vi "SubVI_Prescan Trace.vi"(0 "VISA in":refnum<visa-resource-name>, 1 "Cable 1":T5, 2 "Cable 2":T4, 3 "Cable 3":T3, 5 "Antenna":T6, 7 "Attenuator":T2, 9 "Amplifier":T1=enum."10K-2GHz ME813", 11 "error in (no error)":errorcluster, 12 "Trace 2D array input":dbl[][](array[numeric])) -> (4 "VISA out":refnum<visa-resource-name>, 6 "Start Frequency":dbl, 8 "Stop Frequency":dbl, 10 "Corrected amplitude 1D array":dbl[](array[numeric]), 13 "Completed Result Table":dbl[][](array[numeric]), 14 "Corrected System Trace":cluster{dbl[], "x+y":dbl[]}, 15 "error out":errorcluster)   [LabVIEW 2016]
doc: "This VI generate corrected plot of measurement system adding up antenna factor, cable loss, attenuation and amplification along the way."
uses:
  Antenna.ctl
  Cable 1.ctl
  Cable 2.ctl
  Cable 3.ctl
  Attenuator.ctl
  Amplifier.ctl
panel:
  out "AmplifierX_1D array":dbl[](array[numeric])
  out "AmplifierY_1D array":dbl[](array[numeric]) format="%_6g"
  out "AttenuatorX_1D array":dbl[](array[numeric])
  out "AttenuatorY_1D array":dbl[](array[numeric]) format="%_6g"
  out "Cable3X_1D array":dbl[](array[numeric])
  out "Cable3Y_1D array":dbl[](array[numeric]) format="%_6g"
  out "Cable2X_1D array":dbl[](array[numeric])
  out "Cable2Y_1D array":dbl[](array[numeric]) format="%_6g"
  out "Cable1Y_1D array":dbl[](array[numeric]) format="%_6g"
  out "Cable1X_1D array":dbl[](array[numeric])
  out "Antenna X 1D array":dbl[](array[numeric])
  out "Antenna Y 1D array":dbl[](array[numeric]) format="%_6g"
  out "Nuber of Points":i32
  out "XY Graph":cluster{dbl[], "x+y":dbl[]}(graph)
  out "Corrected 2D array":dbl[][](array[numeric])
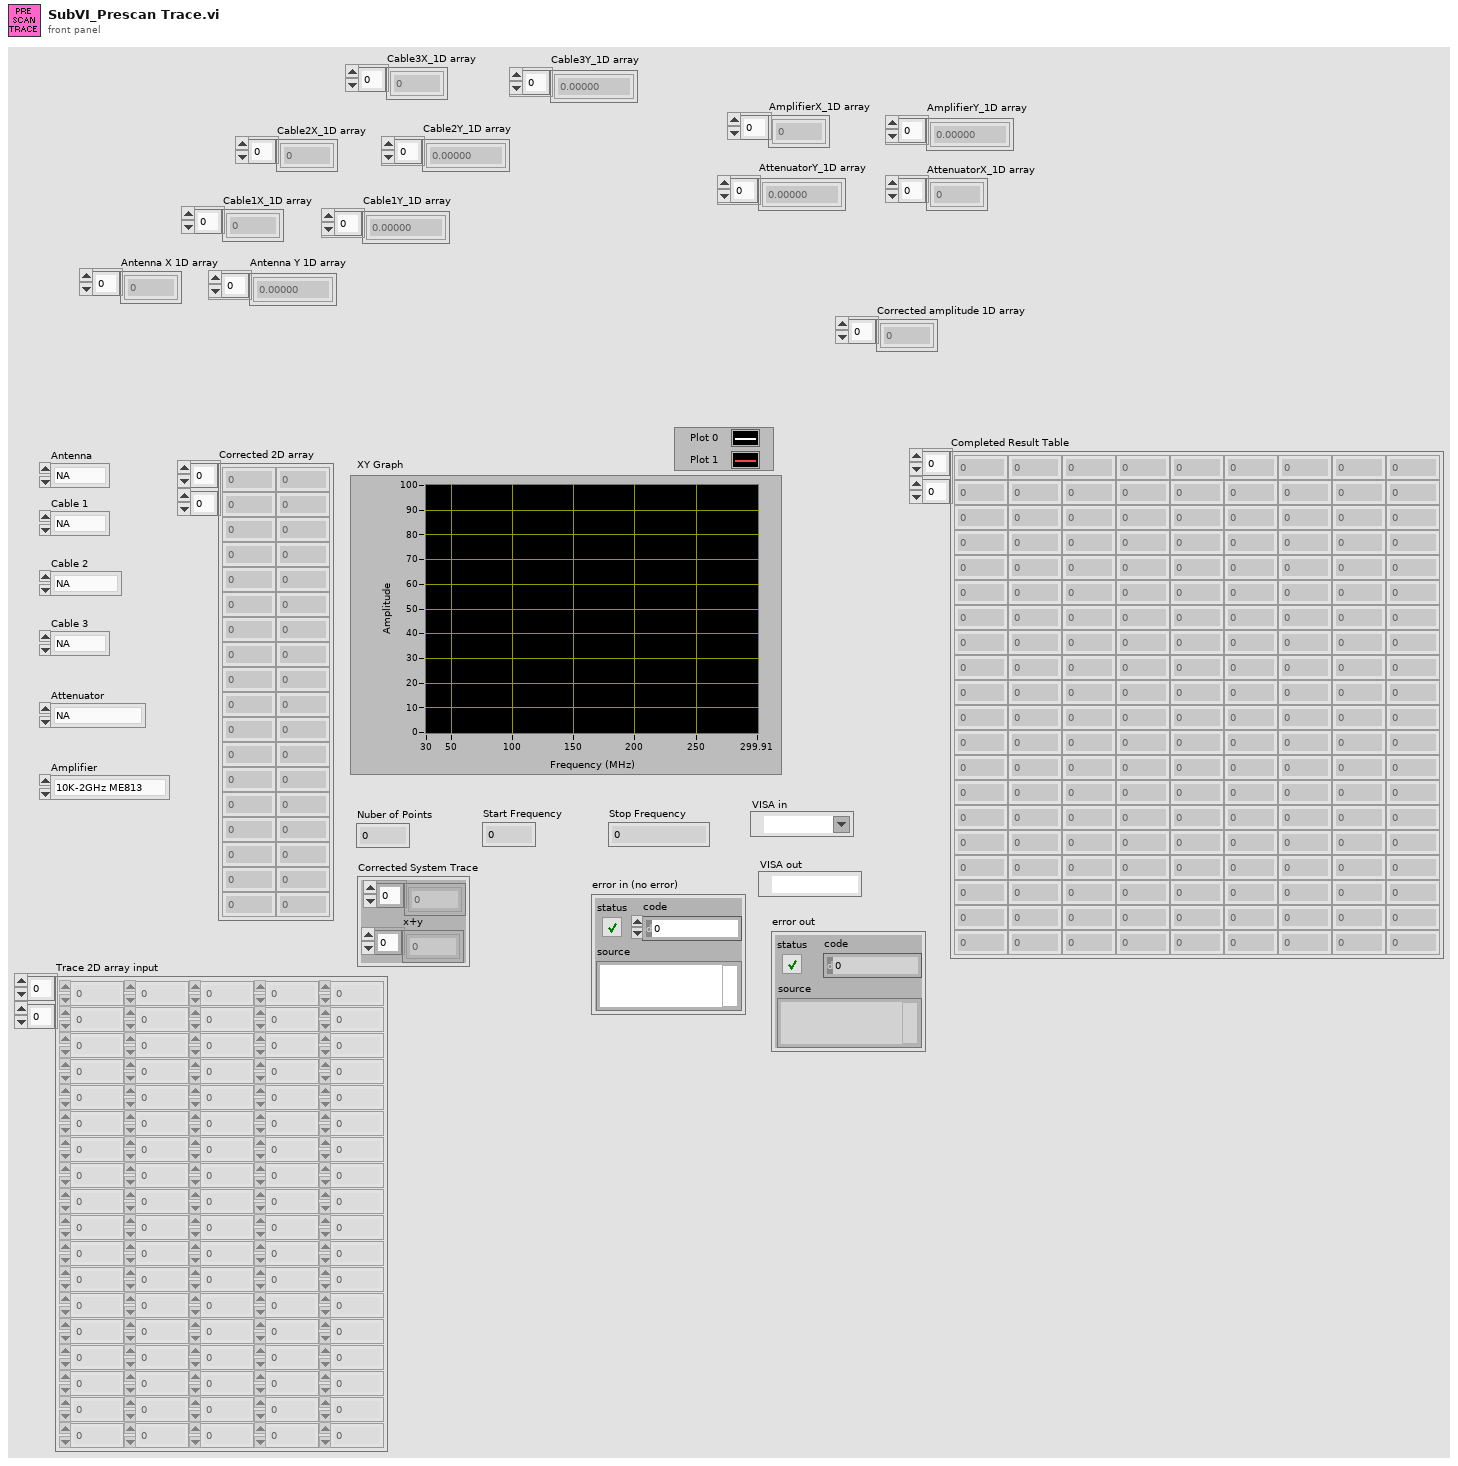
[diagram p1: front panel]
types:
  T1 = typedef "Amplifier.ctl" = enum16{"NA", "10K-2GHz ME813", "500M-18GHz ME1241"}
  T2 = typedef "Attenuator.ctl" = enum16{"NA", "6dB-ME811"}
  T3 = typedef "Cable 3.ctl" = enum16{"NA", "ME1244", "ME1245", "ME1249"}
  T4 = typedef "Cable 2.ctl" = enum16{"NA", "ME1244", "ME1245", "ME1249"}
  T5 = typedef "Cable 1.ctl" = enum16{"NA", "ME1244", "ME1245", "ME1249"}
  T6 = typedef "Antenna.ctl" = enum16{"NA", "ME828 Biconical", "ME1284 Periodical"}
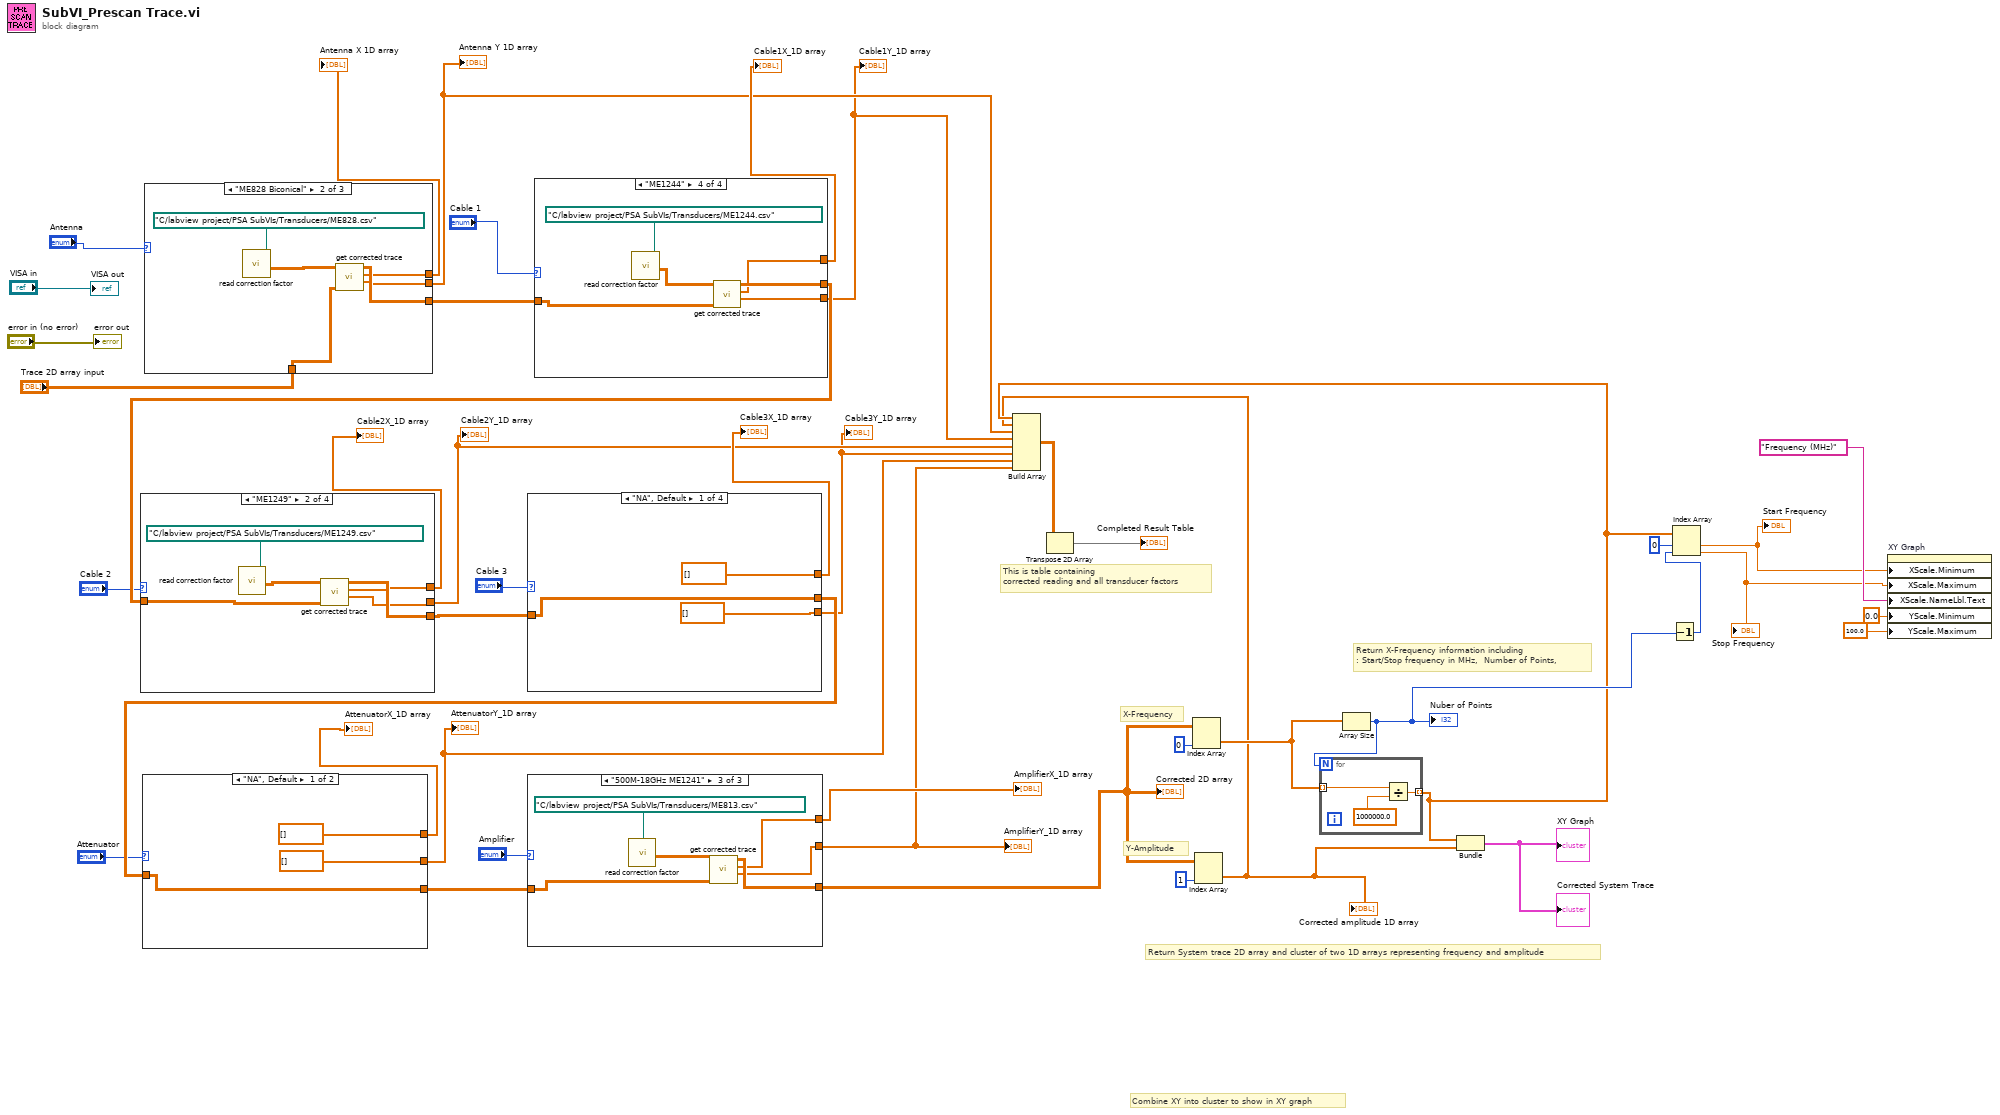
[diagram p0: block diagram]
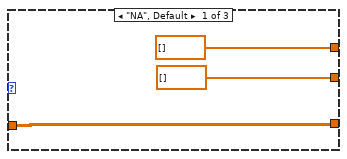
[diagram p2: hidden frame]
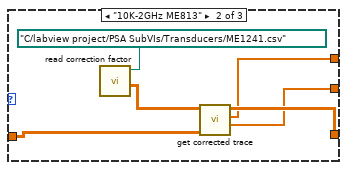
[diagram p3: hidden frame]
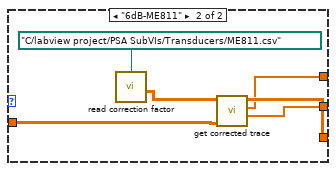
[diagram p4: hidden frame]
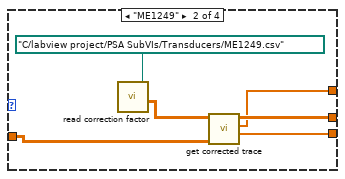
[diagram p5: hidden frame]
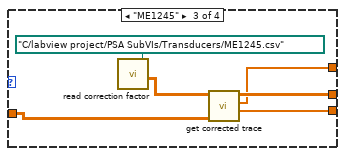
[diagram p6: hidden frame]
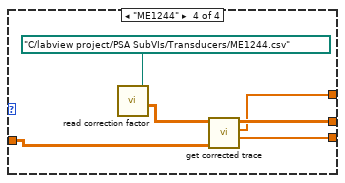
[diagram p7: hidden frame]
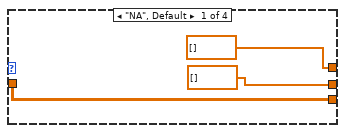
[diagram p8: hidden frame]
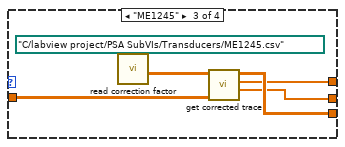
[diagram p9: hidden frame]
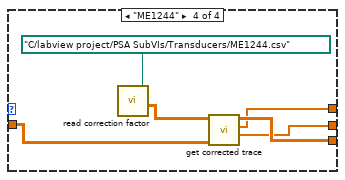
[diagram p10: hidden frame]
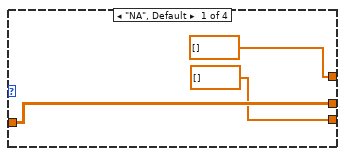
[diagram p11: hidden frame]
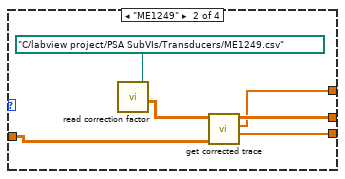
[diagram p12: hidden frame]
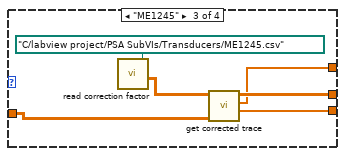
[diagram p13: hidden frame]
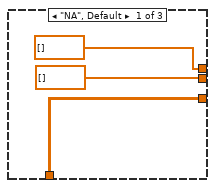
[diagram p14: hidden frame]
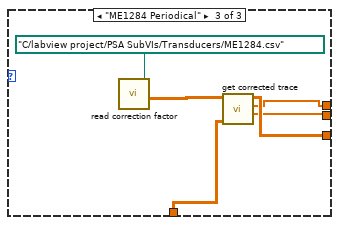
[diagram p15: hidden frame]
diagram:
  # "This is table containing \ncorrected reading and all transducer factors"
  # "Return System trace 2D array and cluster of two 1D arrays representing frequency and amplitude"
  # "Combine XY into cluster to show in XY graph"
  # "Return X-Frequency information including\n: Start/Stop frequency in MHz,  Number of Points,"
  # "Y-Amplitude"
  # "X-Frequency"
  n1 = case shown="\"ME828 Biconical\"" "Antenna" {
    tunnel: "Trace 2D array input" -> [w46 w49 w55]
    tunnel: [w46 w50 w56] -> w43
    tunnel: [dbl[] [] ("xi used") w48 w54] -> w17
    tunnel: [dbl[] [] ("xi used") w47 w53] -> w7
    frame "NA", Default {
    }
    frame "ME828 Biconical" {
      n2 = call "read correction factor.vi"("Path"=path "C:/labview project/PSA SubVIs/Transducers/ME828.csv") -> ("Output Array"=w52:dbl[][])  [unwired: 7 in, 3 out]
      n3 = call "get corrected trace.vi"("Trace 2D array"=w49, "Transducer 2D array"=w52) -> ("yi"=w47:dbl[], "xi used"=w48:dbl[], "x+y"=w50:dbl[][])  [unwired: 7 in]
    }
    frame "ME1284 Periodical" {
      n4 = call "read correction factor.vi"("Path"=path "C:/labview project/PSA SubVIs/Transducers/ME1284.csv") -> ("Output Array"=w58:dbl[][])  [unwired: 7 in, 3 out]
      n5 = call "get corrected trace.vi"("Trace 2D array"=w55, "Transducer 2D array"=w58) -> ("yi"=w53:dbl[], "xi used"=w54:dbl[], "x+y"=w56:dbl[][])  [unwired: 7 in]
    }
  }
  "Antenna Y 1D array" <- w7
  "Antenna X 1D array" <- w17
  n6 = case shown="\"ME1244\"" "Cable 1" {
    tunnel: w43 -> [w61 w65 w71 w77]
    tunnel: [w61 w64 w70 w76] -> w42
    tunnel: [dbl[] [] ("xi used") w63 w69 w75] -> w16
    tunnel: [dbl[] [] ("xi used") w62 w68 w74] -> w6
    frame "NA", Default {
    }
    frame "ME1249" {
      n7 = call "read correction factor.vi"("Path"=path "C:/labview project/PSA SubVIs/Transducers/ME1249.csv") -> ("Output Array"=w66:dbl[][])  [unwired: 7 in, 3 out]
      n8 = call "get corrected trace.vi"("Trace 2D array"=w65, "Transducer 2D array"=w66) -> ("yi"=w62:dbl[], "xi used"=w63:dbl[], "x+y"=w64:dbl[][])  [unwired: 7 in]
    }
    frame "ME1245" {
      n9 = call "read correction factor.vi"("Path"=path "C:/labview project/PSA SubVIs/Transducers/ME1245.csv") -> ("Output Array"=w72:dbl[][])  [unwired: 7 in, 3 out]
      n10 = call "get corrected trace.vi"("Trace 2D array"=w71, "Transducer 2D array"=w72) -> ("yi"=w68:dbl[], "xi used"=w69:dbl[], "x+y"=w70:dbl[][])  [unwired: 7 in]
    }
    frame "ME1244" {
      n11 = call "read correction factor.vi"("Path"=path "C:/labview project/PSA SubVIs/Transducers/ME1244.csv") -> ("Output Array"=w78:dbl[][])  [unwired: 7 in, 3 out]
      n12 = call "get corrected trace.vi"("Trace 2D array"=w77, "Transducer 2D array"=w78) -> ("yi"=w74:dbl[], "xi used"=w75:dbl[], "x+y"=w76:dbl[][])  [unwired: 7 in]
    }
  }
  "Cable1X_1D array" <- w16
  "Cable1Y_1D array" <- w6
  n13 = case shown="\"ME1249\"" "Cable 2" {
    tunnel: w42 -> [w82 w86 w92 w98]
    tunnel: [w82 w85 w91 w97] -> w41
    tunnel: [dbl[] [] ("xi used") w84 w90 w96] -> w15
    tunnel: [dbl[] [] ("xi used") w83 w89 w95] -> w5
    frame "NA", Default {
    }
    frame "ME1249" {
      n14 = call "read correction factor.vi"("Path"=path "C:/labview project/PSA SubVIs/Transducers/ME1249.csv") -> ("Output Array"=w87:dbl[][])  [unwired: 7 in, 3 out]
      n15 = call "get corrected trace.vi"("Trace 2D array"=w86, "Transducer 2D array"=w87) -> ("yi"=w83:dbl[], "xi used"=w84:dbl[], "x+y"=w85:dbl[][])  [unwired: 7 in]
    }
    frame "ME1245" {
      n16 = call "read correction factor.vi"("Path"=path "C:/labview project/PSA SubVIs/Transducers/ME1245.csv") -> ("Output Array"=w93:dbl[][])  [unwired: 7 in, 3 out]
      n17 = call "get corrected trace.vi"("Trace 2D array"=w92, "Transducer 2D array"=w93) -> ("yi"=w89:dbl[], "xi used"=w90:dbl[], "x+y"=w91:dbl[][])  [unwired: 7 in]
    }
    frame "ME1244" {
      n18 = call "read correction factor.vi"("Path"=path "C:/labview project/PSA SubVIs/Transducers/ME1244.csv") -> ("Output Array"=w99:dbl[][])  [unwired: 7 in, 3 out]
      n19 = call "get corrected trace.vi"("Trace 2D array"=w98, "Transducer 2D array"=w99) -> ("yi"=w95:dbl[], "xi used"=w96:dbl[], "x+y"=w97:dbl[][])  [unwired: 7 in]
    }
  }
  "Cable2X_1D array" <- w15
  "Cable2Y_1D array" <- w5
  n20 = case shown="\"NA\", Default" "Cable 3" {
    tunnel: w41 -> [w103 w107 w113 w119]
    tunnel: [w103 w106 w112 w118] -> w40
    tunnel: [dbl[] [] ("xi used") w105 w111 w117] -> w14
    tunnel: [dbl[] [] ("xi used") w104 w110 w116] -> w4
    frame "NA", Default {
    }
    frame "ME1249" {
      n21 = call "read correction factor.vi"("Path"=path "C:/labview project/PSA SubVIs/Transducers/ME1249.csv") -> ("Output Array"=w108:dbl[][])  [unwired: 7 in, 3 out]
      n22 = call "get corrected trace.vi"("Trace 2D array"=w107, "Transducer 2D array"=w108) -> ("yi"=w104:dbl[], "xi used"=w105:dbl[], "x+y"=w106:dbl[][])  [unwired: 7 in]
    }
    frame "ME1245" {
      n23 = call "read correction factor.vi"("Path"=path "C:/labview project/PSA SubVIs/Transducers/ME1245.csv") -> ("Output Array"=w114:dbl[][])  [unwired: 7 in, 3 out]
      n24 = call "get corrected trace.vi"("Trace 2D array"=w113, "Transducer 2D array"=w114) -> ("yi"=w110:dbl[], "xi used"=w111:dbl[], "x+y"=w112:dbl[][])  [unwired: 7 in]
    }
    frame "ME1244" {
      n25 = call "read correction factor.vi"("Path"=path "C:/labview project/PSA SubVIs/Transducers/ME1244.csv") -> ("Output Array"=w120:dbl[][])  [unwired: 7 in, 3 out]
      n26 = call "get corrected trace.vi"("Trace 2D array"=w119, "Transducer 2D array"=w120) -> ("yi"=w116:dbl[], "xi used"=w117:dbl[], "x+y"=w118:dbl[][])  [unwired: 7 in]
    }
  }
  "Cable3X_1D array" <- w14
  "Cable3Y_1D array" <- w4
  n27 = case shown="\"NA\", Default" "Attenuator" {
    tunnel: w40 -> [w124 w128]
    tunnel: [w124 w127] -> w39
    tunnel: [dbl[] [] ("xi used") w126] -> w13
    tunnel: [dbl[] [] ("xi used") w125] -> w3
    frame "NA", Default {
    }
    frame "6dB-ME811" {
      n28 = call "read correction factor.vi"("Path"=path "C:/labview project/PSA SubVIs/Transducers/ME811.csv") -> ("Output Array"=w129:dbl[][])  [unwired: 7 in, 3 out]
      n29 = call "get corrected trace.vi"("Trace 2D array"=w128, "Transducer 2D array"=w129) -> ("yi"=w125:dbl[], "xi used"=w126:dbl[], "x+y"=w127:dbl[][])  [unwired: 7 in]
    }
  }
  "AttenuatorX_1D array" <- w13
  "AttenuatorY_1D array" <- w3
  n30 = case shown="\"500M-18GHz ME1241\"" "Amplifier" {
    tunnel: w39 -> [w133 w137 w143]
    tunnel: [w133 w136 w142] -> w10
    tunnel: [dbl[] [] ("xi used") w135 w141] -> w12
    tunnel: [dbl[] [] ("xi used") w134 w140] -> w2
    frame "NA", Default {
    }
    frame "10K-2GHz ME813" {
      n31 = call "read correction factor.vi"("Path"=path "C:/labview project/PSA SubVIs/Transducers/ME1241.csv") -> ("Output Array"=w138:dbl[][])  [unwired: 7 in, 3 out]
      n32 = call "get corrected trace.vi"("Trace 2D array"=w137, "Transducer 2D array"=w138) -> ("yi"=w134:dbl[], "xi used"=w135:dbl[], "x+y"=w136:dbl[][])  [unwired: 7 in]
    }
    frame "500M-18GHz ME1241" {
      n33 = call "read correction factor.vi"("Path"=path "C:/labview project/PSA SubVIs/Transducers/ME813.csv") -> ("Output Array"=w144:dbl[][])  [unwired: 7 in, 3 out]
      n34 = call "get corrected trace.vi"("Trace 2D array"=w143, "Transducer 2D array"=w144) -> ("yi"=w140:dbl[], "xi used"=w141:dbl[], "x+y"=w142:dbl[][])  [unwired: 7 in]
    }
  }
  "Corrected 2D array" <- w10
  "AmplifierX_1D array" <- w12
  "AmplifierY_1D array" <- w2
  n35 = Index Array(array=w10, index (col)=0 ("disabled index (col)")) -> (element=w31:dbl[])  [unwired: 1 in]
  n36 = Index Array(array=w10, index (col)=1 ("disabled index (col)")) -> (element=w8:dbl[])  [unwired: 1 in]
  "Corrected amplitude 1D array" <- w8
  n37 = Array Size(array=w31) -> (size(s)=w30:i32)
  "Nuber of Points" <- w30
  n38 = for {
    N: w30 -> [_]
    tunnel: w31 -> [w147] mode=indexing
    tunnel: [w146] -> w9 mode=indexing
    n39 = Divide(x=w147, y=1000000.0) -> (x/y=w146:dbl)
  }
  n40 = Build Array(w9, w8, w7, w6, w5, w4, w3, w2) -> (w11:dbl[][])
  n41 = Transpose 2D Array(2D array=w11) -> (transposed array=→"Completed Result Table":dbl[][])
  n42 = Bundle(w9, "x+y"=w8) -> (→"XY Graph" →"Corrected System Trace":cluster{dbl[], "x+y":dbl[]})  [unwired: 1 in]
  n43 = Decrement(x=w30) -> (x-1=w35:i32)
  n44 = Index Array(array=w9, index #1=0 ("index"), index #2=w35) -> (element #1=w33:dbl, element #2=w32:dbl)
  "Start Frequency" <- w33
  "Stop Frequency" <- w32
  n45 = property on="XY Graph" class="XYGraph (strict)"("XScale.Minimum"=w33, "XScale.Maximum"=w32, "XScale.NameLbl.Text"="Frequency (MHz)" ("X Scale.Unit Label.Text"), "YScale.Minimum"=0.0 ("Y Scale.Range:Minimum"), "YScale.Maximum"=100.0 ("Y Scale.Range:Maximum")) -> ()  [unwired: 2 in, 2 out]
  "VISA out" <- "VISA in"
  "error out" <- "error in (no error)"
